vi "工程系数变换.vi"(11 "编码器工程量转换":cluster{"编码器计数值":dbl, "工程计量值":dbl}={"编码器计数值"=1.0, "工程计量值"=1.0}) -> (3 "工程变换系数":dbl)   [LabVIEW 2016, in "elevator.lvlib"]
uses:
  elevator.lvlib
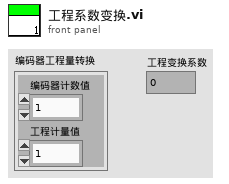
[diagram p1: front panel]
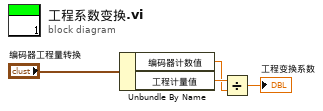
[diagram p0: block diagram]
diagram:
  n1 = Unbundle By Name("编码器工程量转换") -> ("编码器计数值"=w1:dbl, "工程计量值"=w2:dbl)
  n2 = Divide(x=w2, y=w1) -> (x/y=→"工程变换系数":dbl)
